vi "AnalyzeSignalTest-2.vi"() -> ()   [LabVIEW 2019]
uses:
  VibrationDiagnosisDesktopApp/mainVIs/DialogsVIs/AnalysisSettings.ctl
  MobileAnalyzer/mainVIs/analyzeAccelerationDataVIs/calculateFaultIndicatorsVIs/Thresholds.ctl
  MobileAnalyzer/mainVIs/analyzeAccelerationDataVIs/calculateFaultIndicatorsVIs/FaultParameter.ctl
  MobileAnalyzer/mainVIs/aquireAccelerationDataVIs/Accelerometer.ctl
  <vilib>/Waveform/WDTOps.llb/WDT Waveform Duration DBL.vi
panel:
  out "rzędy":T1(graph)
  out "FFT":cluster{"f0":dbl, "df":dbl, "real part":dbl[]}[](graph)
  in  "AnalysisSettings":T2={"Fault Thresholds"={"Parameters labels"=[], "Parameters thresholds"=[], "Freqs and thresholds"=[], "Orders and thresholds"=[]}, "Analysis series name"="Analiza", "Save data analysis?"=TRUE, "F-Band Size"=20, "OrderAnalysis?"=TRUE, "Accelerometer"=enum."MMA7351", "fs [Hz]"=5120.0, "Pulse per revolution"=4, "FFT-Parameters"={"averaging mode"=enum."RMS averaging", "weighting mode"=enum."Linear", "number of averages"=1000}, "O-WindowPowerSpectrum"=1, "O-SpectrumAveraging"=enum."RMS averaging", "O-MaxOrder"=32.0, "O-Resolution"=0.1, "O-BandSize"=0.0, "FrameLength [s]"=1.0, "Aq.FrameLength [ms]"=1000, "FilterOrder"=32, "Sensitivity [V/g]"=[1.0, 1.0, 1.0]}
  in  "STOP":bool
  out "tacho":waveform(dbl)(graph)
  out "acc":waveform(dbl)[](graph)
  in  "sciezka":path
  out "Rotational speed [RPM]":dbl format="%0.2f"
  # "2"
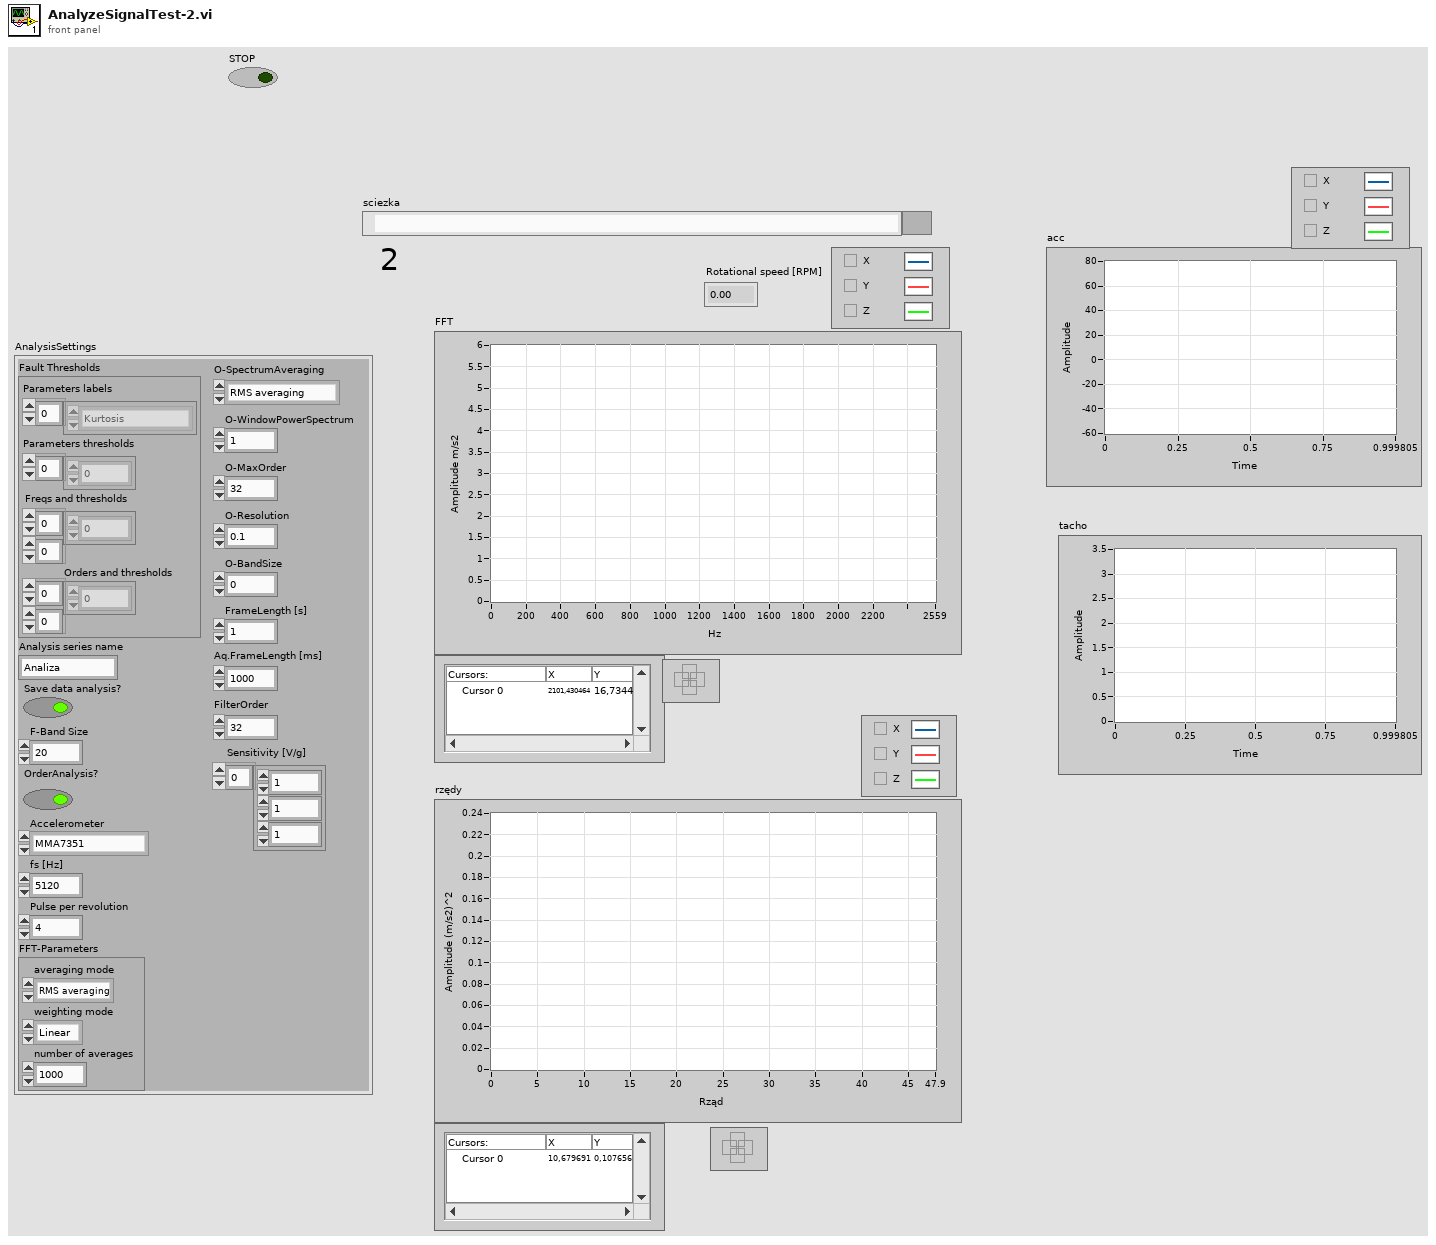
[diagram p1: front panel]
types:
  T1 = cluster{"order 0":dbl, "delta order":dbl, "magnitude":dbl[]}[]
  T2 = typedef "AnalysisSettings.ctl" = cluster{"Fault Thresholds":T3, "Analysis series name":string, "Save data analysis?":bool, "F-Band Size":i32, "OrderAnalysis?":bool, "Accelerometer":T5, "fs [Hz]":dbl, "Pulse per revolution":u16, "FFT-Parameters":cluster{"averaging mode":enum16{"No averaging", "Vector averaging", "RMS averaging", "Peak hold"}, "weighting mode":enum16{"Linear", "Exponential"}, "number of averages":u32}, "O-WindowPowerSpectrum":u32, "O-SpectrumAveraging":enum16{"No averaging", "Vector averaging", "RMS averaging", "Peak hold"}, "O-MaxOrder":dbl, "O-Resolution":dbl, "O-BandSize":dbl, "FrameLength [s]":dbl, "Aq.FrameLength [ms]":i64, "FilterOrder":i32, "Sensitivity [V/g]":dbl[]}
  T3 = typedef "Thresholds.ctl" = cluster{"Parameters labels":T4[], "Parameters thresholds":dbl[], "Freqs and thresholds":dbl[][], "Orders and thresholds":dbl[][]}
  T4 = typedef "FaultParameter.ctl" = enum16{"Kurtosis", "RMS", "Crest factor"}
  T5 = typedef "Accelerometer.ctl" = enum16{"None", "MPU6050", "MMA7351"}
  T6 = enum16{"open", "open or create", "create or replace", "create", "open (read-only)"}
  T7 = typedef "AccelerationDataFrames.ctl" = cluster{"AccelerationData":waveform(dbl)[], "Amplitudes":cluster{"f0":dbl, "df":dbl, "real part":dbl[]}[], "Phases":cluster{"f0":dbl, "df":dbl, "imaginary part":dbl[]}[]}
  T8 = typedef "svc_Spectrum Info.ctl" = cluster{"channel name":string, "description":string, "x-axis units":T9, "spectral info":cluster{"spectrum type":T10, "linear/dB":enum16{"linear", "dB"}, "window":u16, "window size":i32, "FFT size":i32}, "engineering units":T11, "custom label":string, "dB reference [EU]":dbl, "peak units":enum16{"rms", "peak", "peak-peak"}, "weighting filter":T12, "spectral density?":bool, "unit label":string, "spectrum skewed?":bool, "complimentary spectrum units":T13}
  T9 = typedef "svc_X-Axis Units.ctl" = u16
  T10 = typedef "svc_Spectrum Type.ctl" = enum16{"FFT Spectrum [complex]", "Amplitude [Magnitude]", "Power [Magnitude^2]", "Cross Spectrum [complex]", "Frequency Response [Complex]"}
  T11 = typedef "svc_Engineering Units Text Ring.ctl" = u16
  T12 = typedef "svc_Weighting Filter Text Ring.ctl" = u16
  T13 = typedef "svc_Complimentary Spectrum Units.ctl" = enum16{"none", "radians", "degrees", "cycles", "imaginary"}
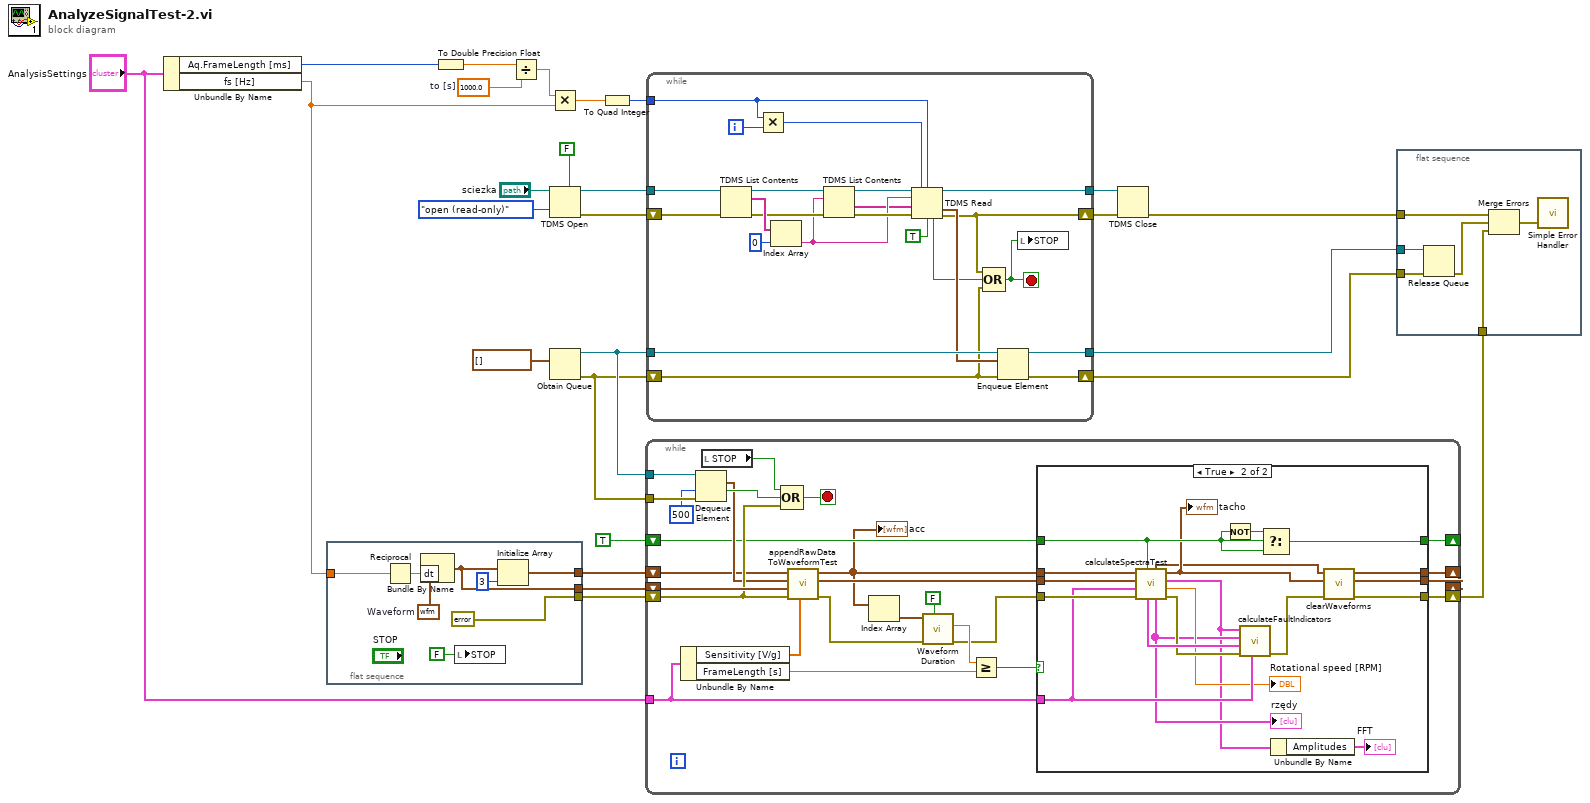
[diagram p0: block diagram]
diagram:
  w17 = 1000.0  # to [s]
  n1 = Unbundle By Name("AnalysisSettings") -> ("Aq.FrameLength [ms]"=w25:i64, "fs [Hz]"=w1:dbl)
  n2 = flat-sequence {
    tunnel: [w31] -> w23
    tunnel: [w30] -> w22
    tunnel: w1 -> [w29]
    tunnel: [errorcluster {"status"=FALSE, "code"=0, "source"=""} ("ErrorOut")] -> w6
    frame #0 {
      w32 = waveform(dbl) {"t0"=timestamp(0 s since 1904-01-01), "dt"=0.0, "Y"=[]}  # Waveform
      n3 = Reciprocal(x=w29) -> (1/x=w34:dbl)
      n4 = Bundle By Name(cluster=w32, "dt"=w34) -> (w30:waveform(dbl))
      n5 = local write "STOP"(FALSE ("STOP")) -> ()
      n6 = Initialize Array(w30, 3 ("dimension size")) -> (w31:waveform(dbl)[])
    }
  }
  n7 = To Double Precision Float(number=w25) -> (double precision float=w4:dbl)
  n8 = Divide(x=w4, y=w17) -> (x/y=w15:dbl)
  n9 = Multiply(x=w15, y=w1) -> (x*y=w16:dbl)
  n10 = TDMS Open(5:FALSE ("create index file? (T)"), 10:T6."open (read-only)" ("operation (0:open)"), 11:"sciezka") -> (0:w19:errorcluster, 3:w20:refnum<k34>)  [unwired: 4 in]
  n11 = Obtain Queue(element data type=waveform(dbl)[] [] ("data")) -> (queue out=w12:refnum<queue>, error out=w11:errorcluster)  [unwired: 4 in, 1 out]
  n12 = To Quad Integer(1:w16) -> (0:w18:i64)
  n13 = while {
    shift-right: [w53] -> _
    shift-left: w23 -> [w36]
    shift-right: [w52] -> _
    shift-left: w22 -> [w54]
    shift-right: [w51] -> w9
    shift-left: w6 -> [w48]
    tunnel: w12 -> [w50]
    tunnel: w11 -> [w49]
    tunnel: "AnalysisSettings" -> [w41]
    shift-right: [w38] -> _
    shift-left: TRUE ("restart averaging (F)") -> [w39]
    stop <- w47 stop-if-true
    n14 = Unbundle By Name(w41) -> ("Sensitivity [V/g]"=w37:dbl[], "FrameLength [s]"=w42:dbl)
    n15 = Dequeue Element(queue=w50, timeout in ms (-1)=500, error in (no error)=w49) -> (element=w40:waveform(dbl)[], timed out?=w46:bool)  [unwired: 2 out]
    n16 = local read "STOP"() -> (w45:bool)
    n17 = Compound Arithmetic op=OR(w45, w46, w48) -> (w47:bool)
    n18 = call "appendRawDataToWaveformTest.vi"("Czułości [V/g]"=w37, "ErrorIn"=w48, "Tacho signal In"=w54, "RawAccData"=w40, "AccelerationDataIn"=w36) -> ("ErrorOut"=w55:errorcluster, "Tacho signal Out"=w56:waveform(dbl), "AccelerationDataOut"=w35:waveform(dbl)[])  [unwired: 4 in]
    "acc" <- w35
    n19 = Index Array(array=w35) -> (element=w60:waveform(dbl))  [unwired: 1 in]
    n20 = call-poly <vilib>:"Waveform Duration.vi"("open interval? (T)"=FALSE, "error in (no error)"=w55, "waveform in"=w60) -> ("error out"=w57:errorcluster, "duration"=w59:dbl)  [unwired: 6 in, 1 out]
    n21 = Greater Or Equal?(x=w59, y=w42) -> (x >= y?=w58:bool)
    n22 = case shown="True" w58 {
      tunnel: w57 -> [w64 w78]
      tunnel: w35 -> [w63 w79]
      tunnel: w56 -> [w62 w77]
      tunnel: [w64 w83] -> w51
      tunnel: [w63 w82] -> w53
      tunnel: [w62 w81] -> w52
      tunnel: w41 -> [_ w76]
      tunnel: w39 -> [w61 w68]
      tunnel: [w61 w70] -> w38
      frame False {
      }
      frame True {
        n23 = call "calculateSpectraTest.vi"("Reset?"=w68, "ErrorIn"=w78, "AnalysisSettings"=w76, "Tacho signal In"=w77, "AccelerationDataIn"=w79) -> ("ErrorOut"=w74:errorcluster, "Rotational speed [RPM]"=→"Rotational speed [RPM]":dbl, "AccelerationDataFrames"=w71:T7, "Tacho signal out"=w66:waveform(dbl), "order power spectra"=w72:T1, "AccelerationDataOut"=w65:waveform(dbl)[], "spectrum info"=w75:T8[])
        "tacho" <- w66
        "rzędy" <- w72
        n24 = Not(x=w68) -> (.not. x?=w69:bool)
        n25 = call "calculateFaultIndicators.vi"("AnalysisSettings"=w76, "ErrorIn"=w74, "spectrum info"=w75, "order power spectra"=w72, "AccelerationDataFrames"=w71) -> ("ErrorOut"=w80:errorcluster)  [unwired: 4 in, 2 out]
        n26 = Select(t=w69, s=w68, f=w68) -> (s? t:f=w70:bool)
        n27 = Unbundle By Name(w71) -> ("Amplitudes"=→"FFT":cluster{"f0":dbl, "df":dbl, "real part":dbl[]}[])
        n28 = call "clearWaveforms.vi"("ErrorIn"=w80, "Tacho signal In"=w66, "AccelerationDataIn"=w65) -> ("ErrorOut"=w83:errorcluster, "Tacho signal Out"=w81:waveform(dbl), "AccelerationDataOut"=w82:waveform(dbl)[])  [unwired: 6 in]
      }
    }
  }
  n29 = while {
    tunnel: w12 -> [w100]
    tunnel: w20 -> [w106]
    tunnel: w18 -> [w102]
    tunnel: [w101] -> w14
    shift-right: [w94] -> w13
    shift-left: w19 -> [w105]
    tunnel: [w98] -> w7
    shift-right: [w97] -> w8
    shift-left: w11 -> [w96]
    i -> [w104]
    stop <- w93 stop-if-true
    n30 = TDMS List Contents(4:w105, 7:w106) -> (0:w87:errorcluster, 2:w91:string[], 3:w89:refnum<k34>)  [unwired: 1 in, 1 out]
    n31 = Multiply(x=w102, y=w104) -> (x*y=w103:i64)
    n32 = Index Array(array=w91, index=0) -> (element=w85:string)
    n33 = TDMS List Contents(4:w87, 6:w85, 7:w89) -> (0:w86:errorcluster, 1:w84:string[], 3:w88:refnum<k34>)  [unwired: 1 out]
    n34 = TDMS Read(0:w88, 1:w103, 2:w102, 5:w85, 7:w84, 11:w86, 13:TRUE ("return channels in file order? (F)")) -> (4:w101:refnum<k34>, 10:w99:waveform(dbl)[], 14:w95:bool, 15:w94:errorcluster)  [unwired: 1 in, 2 out]
    n35 = Compound Arithmetic op=OR(w94, w95, w96) -> (w93:bool)
    n36 = Enqueue Element(queue=w100, element=w99, error in (no error)=w96) -> (queue out=w98:refnum<queue>, error out=w97:errorcluster)  [unwired: 1 in, 1 out]
    n37 = local write "STOP"(w93) -> ()
  }
  n38 = TDMS Close(8:w13, 11:w14) -> (0:w10:errorcluster)  [unwired: 1 out]
  n39 = flat-sequence {
    tunnel: w10 -> [w112]
    tunnel: w9 -> [w111]
    tunnel: w8 -> [w110]
    tunnel: w7 -> [w109]
    frame #0 {
      n40 = Release Queue(queue=w109, error in (no error)=w110) -> (error out=w108:errorcluster)  [unwired: 1 in, 2 out]
      n41 = Merge Errors(w112, w108, w111) -> (w107:errorcluster)
      n42 = call <vilib>:"Simple Error Handler.vi"("error in (no error)"=w107) -> ()  [unwired: 4 in, 5 out]
    }
  }
